vi "IV(H)_2devices_DC_temperature sweep_BF_LD-400_K6221_K2182A_PK.vi"() -> ()   [LabVIEW 2016]
uses:
  <vilib>/Math Plots/2D Math Plots/2D Compass/2D Compass XCtrl/2D Compass.xctl
  <vilib>/Math Plots/2D Math Plots/2D Compass/2D Compass Datatype/2D Compass Datatype.lvclass
  <vilib>/Math Plots/2D Math Plots/2D Compass/2D Compass Datatype/Public/Plot Helper (Vector).vi
  Labview Drivers/Keithley 622x LV 2009/Keithley 622x.lvlib
panel:
  out "data 2":dbl[](array[numeric])=[0.5999981386233562, 330.0003030452058, -2e-06, -1.74783916e-05, 8.739195800000001, 14115.23]
  out "File path 2":path=path "D:/Pranava/Data/PtTe2/29-10-2022/002/025_29-10-2022_002_DevD2_I_39-36_V_42-41_DC_IV(H)_baseT_[450mT_to_-650mT]_IP_[150deg]_10mT_steps.dat"
  in  "Measure two devices?":bool
  out "2D Compass":refnum<class "2D Plot Datatype.lvclass">[](xcontrol)
  in  "Number Averaging":i32=1
  in  "Tab Control":enum32{"Device 1", "Device 2"}(tab)=enum."Device 2"
  out "V vs I":cluster{dbl, "Field Reading":dbl}[](graph)=[{0.0, "Field Reading"=4.40241798e-08}, {2e-08, "Field Reading"=1.23783257e-07}, {4e-08, "Field Reading"=3.02986118e-07}, {6e-08, "Field Reading"=5.49519534e-07}, {8e-08, "Field Reading"=7.0386157e-07}, {1e-07, "Field Reading"=8.50435e-07}, {1.2e-07, "Field Reading"=1.09593255e-06}, {1.4e-07, "Field Reading"=1.21350074e-06}, {1.6e-07, "Field Reading"=1.39529319e-06}, {1.8e-07, "Field Reading"=1.54134866e-06}, {2e-07, "Field Reading"=1.75991058e-06}, {2.2e-07, "Field Reading"=1.91891414e-06}, {2.4e-07, "Field Reading"=2.05875441e-06}, {2.6e-07, "Field Reading"=2.23173979e-06}, {2.8e-07, "Field Reading"=2.36018563e-06}, {3e-07, "Field Reading"=2.64452742e-06}, {3.2e-07, "Field Reading"=2.75122088e-06}, {3.4e-07, "Field Reading"=2.90763477e-06}, {3.6e-07, "Field Reading"=3.12050268e-06}, {3.8e-07, "Field Reading"=3.23392292e-06}, {4e-07, "Field Reading"=3.48200967e-06}, {4.2e-07, "Field Reading"=3.63013662e-06}, {4.4e-07, "Field Reading"=3.79483537e-06}, {4.6e-07, "Field Reading"=3.94296229e-06}, {4.8e-07, "Field Reading"=4.10869871e-06}, {5e-07, "Field Reading"=4.332443e-06}, {5.2e-07, "Field Reading"=4.44638679e-06}, {5.4e-07, "Field Reading"=4.61160528e-06}, {5.6e-07, "Field Reading"=4.8415635e-06}, {5.8e-07, "Field Reading"=4.99228004e-06}, {6e-07, "Field Reading"=5.17562593e-06}, {6.2e-07, "Field Reading"=5.33774246e-06}, {6.4e-07, "Field Reading"=5.53403662e-06}, {6.6e-07, "Field Reading"=5.65315972e-06}, {6.8e-07, "Field Reading"=5.83340484e-06}, {7e-07, "Field Reading"=6.04161144e-06}, {7.2e-07, "Field Reading"=6.14312511e-06}, {7.4e-07, "Field Reading"=6.37827086e-06}, {7.6e-07, "Field Reading"=6.53727451e-06}, {7.8e-07, "Field Reading"=6.69938572e-06}, {8e-07, "Field Reading"=6.88635475e-06}, {8.2e-07, "Field Reading"=7.02101579e-06}, {8.4e-07, "Field Reading"=7.23699138e-06}, {8.6e-07, "Field Reading"=7.41308471e-06}, {8.8e-07, "Field Reading"=7.58244684e-06}, {9e-07, "Field Reading"=7.74041457e-06}, {9.2e-07, "Field Reading"=7.90562381e-06}, {9.4e-07, "Field Reading"=8.06618106e-06}, {9.6e-07, "Field Reading"=8.2422761e-06}, {9.8e-07, "Field Reading"=8.41162272e-06}, {1e-06, "Field Reading"=8.59082511e-06}, {1.02e-06, "Field Reading"=8.73842623e-06}, {1.04e-06, "Field Reading"=8.94248895e-06}, {1.06e-06, "Field Reading"=9.14240827e-06}, {1.08e-06, "Field Reading"=9.27862314e-06}, {1.1e-06, "Field Reading"=9.47388113e-06}, {1.12e-06, "Field Reading"=9.62770506e-06}, {1.14e-06, "Field Reading"=9.81261485e-06}, {1.16e-06, "Field Reading"=9.94365015e-06}, {1.18e-06, "Field Reading"=1.0168948e-05}, {1.2e-06, "Field Reading"=1.03238199e-05}, {1.22e-06, "Field Reading"=1.05263292e-05}, {1.24e-06, "Field Reading"=1.0654257e-05}, {1.26e-06, "Field Reading"=1.08365675e-05}, {1.28e-06, "Field Reading"=1.09608698e-05}, {1.3e-06, "Field Reading"=1.11291959e-05}, {1.32e-06, "Field Reading"=1.13104759e-05}, {1.34e-06, "Field Reading"=1.14658539e-05}, {1.36e-06, "Field Reading"=1.17056539e-05}, {1.38e-06, "Field Reading"=1.1880715e-05}, {1.4e-06, "Field Reading"=1.20252166e-05}, {1.42e-06, "Field Reading"=1.22121882e-05}, {1.44e-06, "Field Reading"=1.23541037e-05}, {1.46e-06, "Field Reading"=1.2493426e-05}, {1.48e-06, "Field Reading"=1.27368517e-05}, {1.5e-06, "Field Reading"=1.28668613e-05}, {1.52e-06, "Field Reading"=1.3010845e-05}, {1.54e-06, "Field Reading"=1.31729562e-05}, {1.56e-06, "Field Reading"=1.34153398e-05}, {1.58e-06, "Field Reading"=1.3541714e-05}, {1.6e-06, "Field Reading"=1.36877694e-05}, {1.62e-06, "Field Reading"=1.38659327e-05}, {1.64e-06, "Field Reading"=1.40705138e-05}, {1.66e-06, "Field Reading"=1.42554137e-05}, {1.68e-06, "Field Reading"=1.43978348e-05}, {1.7e-06, "Field Reading"=1.45537307e-05}, {1.72e-06, "Field Reading"=1.4763491e-05}, {1.74e-06, "Field Reading"=1.49478731e-05}, {1.76e-06, "Field Reading"=1.50571556e-05}, {1.78e-06, "Field Reading"=1.5244645e-05}, {1.8e-06, "Field Reading"=1.54171202e-05}, {1.82e-06, "Field Reading"=1.55590321e-05}, {1.84e-06, "Field Reading"=1.57708642e-05}, {1.86e-06, "Field Reading"=1.59593796e-05}, {1.88e-06, "Field Reading"=1.60826461e-05}, {1.9e-06, "Field Reading"=1.62836016e-05}, {1.92e-06, "Field Reading"=1.64534904e-05}, {1.94e-06, "Field Reading"=1.65871155e-05}, {1.96e-06, "Field Reading"=1.68072344e-05}, {1.98e-06, "Field Reading"=1.69807332e-05}, {2e-06, "Field Reading"=1.71039997e-05}, {2.02e-06, "Field Reading"=1.73298157e-05}, {2.04e-06, "Field Reading"=1.75338777e-05}, {2.06e-06, "Field Reading"=1.76706104e-05}, {2.08e-06, "Field Reading"=1.78063071e-05}, {2.1e-06, "Field Reading"=1.79881126e-05}, {2.12e-06, "Field Reading"=1.81730125e-05}, {2.14e-06, "Field Reading"=1.83542869e-05}, {2.16e-06, "Field Reading"=1.84765118e-05}, {2.18e-06, "Field Reading"=1.86950769e-05}, {2.2e-06, "Field Reading"=1.88804946e-05}, {2.22e-06, "Field Reading"=1.90384784e-05}, {2.24e-06, "Field Reading"=1.91767649e-05}, {2.26e-06, "Field Reading"=1.93580394e-05}, {2.28e-06, "Field Reading"=1.95553725e-05}, {2.3e-06, "Field Reading"=1.97330215e-05}, {2.32e-06, "Field Reading"=1.98827024e-05}, {2.34e-06, "Field Reading"=2.00670785e-05}, {2.36e-06, "Field Reading"=2.02561219e-05}, {2.38e-06, "Field Reading"=2.04550059e-05}, {2.4e-06, "Field Reading"=2.05839566e-05}, {2.42e-06, "Field Reading"=2.07004901e-05}, {2.44e-06, "Field Reading"=2.08941947e-05}, {2.46e-06, "Field Reading"=2.10935914e-05}, {2.48e-06, "Field Reading"=2.12541486e-05}, {2.5e-06, "Field Reading"=2.14209052e-05}, {2.52e-06, "Field Reading"=2.16146097e-05}, {2.54e-06, "Field Reading"=2.18026169e-05}, {2.56e-06, "Field Reading"=2.19916641e-05}, {2.58e-06, "Field Reading"=2.21568827e-05}, {2.6e-06, "Field Reading"=2.23319418e-05}, {2.62e-06, "Field Reading"=2.2459882e-05}, {2.64e-06, "Field Reading"=2.26406384e-05}, {2.66e-06, "Field Reading"=2.28395223e-05}, {2.68e-06, "Field Reading"=2.2994903e-05}, {2.7e-06, "Field Reading"=2.31471734e-05}, {2.72e-06, "Field Reading"=2.32978901e-05}, {2.74e-06, "Field Reading"=2.34921259e-05}, {2.76e-06, "Field Reading"=2.36547549e-05}, {2.78e-06, "Field Reading"=2.38215274e-05}, {2.8e-06, "Field Reading"=2.40152458e-05}, {2.82e-06, "Field Reading"=2.41934127e-05}, {2.84e-06, "Field Reading"=2.43938505e-05}, {2.86e-06, "Field Reading"=2.4514533e-05}, {2.88e-06, "Field Reading"=2.47548513e-05}, {2.9e-06, "Field Reading"=2.48532575e-05}, {2.92e-06, "Field Reading"=2.50619679e-05}, {2.94e-06, "Field Reading"=2.51930034e-05}, {2.96e-06, "Field Reading"=2.5380493e-05}, {2.98e-06, "Field Reading"=2.55322419e-05}, {3e-06, "Field Reading"=2.57492533e-05}, {3e-06, "Field Reading"=2.57720421e-05}, {2e-06, "Field Reading"=1.71412944e-05}, {1e-06, "Field Reading"=8.50279535e-06}, {0.0, "Field Reading"=-1.17576765e-07}, {-2e-08, "Field Reading"=-2.68811351e-07}, {-4e-08, "Field Reading"=-4.69766897e-07}, {-6e-08, "Field Reading"=-6.21518846e-07}, {-8e-08, "Field Reading"=-8.17295154e-07}, {-1e-07, "Field Reading"=-9.41079645e-07}, {-1.2e-07, "Field Reading"=-1.18502315e-06}, {-1.4e-07, "Field Reading"=-1.34454459e-06}, {-1.6e-07, "Field Reading"=-1.46573945e-06}, {-1.8e-07, "Field Reading"=-1.69051911e-06}, {-2e-07, "Field Reading"=-1.82621594e-06}, {-2.2e-07, "Field Reading"=-2.0126696e-06}, {-2.4e-07, "Field Reading"=-2.21776914e-06}, {-2.6e-07, "Field Reading"=-2.35450179e-06}, {-2.8e-07, "Field Reading"=-2.58601504e-06}, {-3e-07, "Field Reading"=-2.69322674e-06}, {-3.2e-07, "Field Reading"=-2.83721031e-06}, {-3.4e-07, "Field Reading"=-3.08995843e-06}, {-3.6e-07, "Field Reading"=-3.19457944e-06}, {-3.8e-07, "Field Reading"=-3.37844337e-06}, {-4e-07, "Field Reading"=-3.57266625e-06}, {-4.2e-07, "Field Reading"=-3.76792448e-06}, {-4.4e-07, "Field Reading"=-3.93469675e-06}, {-4.6e-07, "Field Reading"=-4.04864062e-06}, {-4.8e-07, "Field Reading"=-4.20505435e-06}, {-5e-07, "Field Reading"=-4.46867881e-06}, {-5.2e-07, "Field Reading"=-4.63596869e-06}, {-5.4e-07, "Field Reading"=-4.79238132e-06}, {-5.6e-07, "Field Reading"=-4.99799659e-06}, {-5.8e-07, "Field Reading"=-5.13783554e-06}, {-6e-07, "Field Reading"=-5.31133956e-06}, {-6.2e-07, "Field Reading"=-5.45014278e-06}, {-6.4e-07, "Field Reading"=-5.69460221e-06}, {-6.6e-07, "Field Reading"=-5.77436228e-06}, {-6.8e-07, "Field Reading"=-5.97428035e-06}, {-7e-07, "Field Reading"=-6.12913905e-06}, {-7.2e-07, "Field Reading"=-6.38136727e-06}, {-7.4e-07, "Field Reading"=-6.52534971e-06}, {-7.6e-07, "Field Reading"=-6.63359599e-06}, {-7.8e-07, "Field Reading"=-6.85112346e-06}, {-8e-07, "Field Reading"=-7.07020515e-06}, {-8.2e-07, "Field Reading"=-7.20641881e-06}, {-8.4e-07, "Field Reading"=-7.40167564e-06}, {-8.6e-07, "Field Reading"=-7.54669386e-06}, {-8.8e-07, "Field Reading"=-7.71035741e-06}, {-9e-07, "Field Reading"=-7.89525579e-06}, {-9.2e-07, "Field Reading"=-8.04286623e-06}, {-9.4e-07, "Field Reading"=-8.20031482e-06}, {-9.6e-07, "Field Reading"=-8.37226526e-06}, {-9.8e-07, "Field Reading"=-8.56441587e-06}, {-1e-06, "Field Reading"=-8.75760121e-06}, {-1.02e-06, "Field Reading"=-8.97305724e-06}, {-1.04e-06, "Field Reading"=-9.09994792e-06}, {-1.06e-06, "Field Reading"=-9.267755e-06}, {-1.08e-06, "Field Reading"=-9.48372893e-06}, {-1.1e-06, "Field Reading"=-9.64739249e-06}, {-1.12e-06, "Field Reading"=-9.79396472e-06}, {-1.14e-06, "Field Reading"=-9.97938118e-06}, {-1.16e-06, "Field Reading"=-1.00990192e-05}, {-1.18e-06, "Field Reading"=-1.03647137e-05}, {-1.2e-06, "Field Reading"=-1.04952302e-05}, {-1.22e-06, "Field Reading"=-1.06247112e-05}, {-1.24e-06, "Field Reading"=-1.08479359e-05}, {-1.26e-06, "Field Reading"=-1.10452646e-05}, {-1.28e-06, "Field Reading"=-1.11291712e-05}, {-1.3e-06, "Field Reading"=-1.13979733e-05}, {-1.32e-06, "Field Reading"=-1.15290079e-05}, {-1.34e-06, "Field Reading"=-1.17107996e-05}, {-1.36e-06, "Field Reading"=-1.18584077e-05}, {-1.38e-06, "Field Reading"=-1.2031394e-05}, {-1.4e-06, "Field Reading"=-1.22214705e-05}, {-1.42e-06, "Field Reading"=-1.23742578e-05}, {-1.44e-06, "Field Reading"=-1.25384394e-05}, {-1.46e-06, "Field Reading"=-1.27621798e-05}, {-1.48e-06, "Field Reading"=-1.28792304e-05}, {-1.5e-06, "Field Reading"=-1.30289101e-05}, {-1.52e-06, "Field Reading"=-1.32428105e-05}, {-1.54e-06, "Field Reading"=-1.34660352e-05}, {-1.56e-06, "Field Reading"=-1.35644406e-05}, {-1.58e-06, "Field Reading"=-1.37255157e-05}, {-1.6e-06, "Field Reading"=-1.39409717e-05}, {-1.62e-06, "Field Reading"=-1.41439974e-05}, {-1.64e-06, "Field Reading"=-1.42952297e-05}, {-1.66e-06, "Field Reading"=-1.44941121e-05}, {-1.68e-06, "Field Reading"=-1.45919995e-05}, {-1.7e-06, "Field Reading"=-1.47965808e-05}, {-1.72e-06, "Field Reading"=-1.50275744e-05}, {-1.74e-06, "Field Reading"=-1.51088883e-05}, {-1.76e-06, "Field Reading"=-1.5286534e-05}, {-1.78e-06, "Field Reading"=-1.55475671e-05}, {-1.8e-06, "Field Reading"=-1.56418291e-05}, {-1.82e-06, "Field Reading"=-1.58401957e-05}, {-1.84e-06, "Field Reading"=-1.60354527e-05}, {-1.86e-06, "Field Reading"=-1.61778815e-05}, {-1.88e-06, "Field Reading"=-1.64109433e-05}, {-1.9e-06, "Field Reading"=-1.65114203e-05}, {-1.92e-06, "Field Reading"=-1.67460393e-05}, {-1.94e-06, "Field Reading"=-1.69164354e-05}, {-1.96e-06, "Field Reading"=-1.7107031e-05}, {-1.98e-06, "Field Reading"=-1.72157948e-05}, {-2e-06, "Field Reading"=-1.73789424e-05}, {-2.02e-06, "Field Reading"=-1.7616151e-05}, {-2.04e-06, "Field Reading"=-1.77135205e-05}, {-2.06e-06, "Field Reading"=-1.788599e-05}, {-2.08e-06, "Field Reading"=-1.80781394e-05}, {-2.1e-06, "Field Reading"=-1.82045126e-05}, {-2.12e-06, "Field Reading"=-1.84603712e-05}, {-2.14e-06, "Field Reading"=-1.8589852e-05}, {-2.16e-06, "Field Reading"=-1.87690534e-05}, {-2.18e-06, "Field Reading"=-1.89917572e-05}, {-2.2e-06, "Field Reading"=-1.91388473e-05}, {-2.22e-06, "Field Reading"=-1.93584466e-05}, {-2.24e-06, "Field Reading"=-1.95366097e-05}, {-2.26e-06, "Field Reading"=-1.96655725e-05}, {-2.28e-06, "Field Reading"=-1.98468455e-05}, {-2.3e-06, "Field Reading"=-2.00260392e-05}, {-2.32e-06, "Field Reading"=-2.02104196e-05}, {-2.34e-06, "Field Reading"=-2.03642427e-05}, {-2.36e-06, "Field Reading"=-2.05486354e-05}, {-2.38e-06, "Field Reading"=-2.07009048e-05}, {-2.4e-06, "Field Reading"=-2.08485128e-05}, {-2.42e-06, "Field Reading"=-2.10551707e-05}, {-2.44e-06, "Field Reading"=-2.12468023e-05}, {-2.46e-06, "Field Reading"=-2.14161632e-05}, {-2.48e-06, "Field Reading"=-2.1574128e-05}, {-2.5e-06, "Field Reading"=-2.17181107e-05}, {-2.52e-06, "Field Reading"=-2.18755593e-05}, {-2.54e-06, "Field Reading"=-2.21179489e-05}, {-2.56e-06, "Field Reading"=-2.22878278e-05}, {-2.58e-06, "Field Reading"=-2.246185e-05}, {-2.6e-06, "Field Reading"=-2.26146323e-05}, {-2.62e-06, "Field Reading"=-2.28161044e-05}, {-2.64e-06, "Field Reading"=-2.29424776e-05}, {-2.66e-06, "Field Reading"=-2.30880191e-05}, {-2.68e-06, "Field Reading"=-2.32863837e-05}, {-2.7e-06, "Field Reading"=-2.34681748e-05}, {-2.72e-06, "Field Reading"=-2.36484132e-05}, {-2.74e-06, "Field Reading"=-2.38566183e-05}, {-2.76e-06, "Field Reading"=-2.39985293e-05}, {-2.78e-06, "Field Reading"=-2.41513117e-05}, {-2.8e-06, "Field Reading"=-2.43227442e-05}, {-2.82e-06, "Field Reading"=-2.44646552e-05}, {-2.84e-06, "Field Reading"=-2.46112313e-05}, {-2.86e-06, "Field Reading"=-2.47919865e-05}, {-2.88e-06, "Field Reading"=-2.50271236e-05}, {-2.9e-06, "Field Reading"=-2.51327718e-05}, {-2.92e-06, "Field Reading"=-2.53295825e-05}, {-2.94e-06, "Field Reading"=-2.55269109e-05}, {-2.96e-06, "Field Reading"=-2.57024868e-05}, {-2.98e-06, "Field Reading"=-2.5883242e-05}, {-3e-06, "Field Reading"=-2.59930485e-05}, {-3e-06, "Field Reading"=-2.60981869e-05}, {-2e-06, "Field Reading"=-1.74783916e-05}]
  in  "File name 1":string="027_29-10-2022_002_DevH3_I_46-48_V_45-43_DC_IV(H)_baseT_[-600mT_to_600mT]_IP_[146deg]_5mT_steps"
  in  "From 3":dbl[](array[numeric])=[0.0, 0.00032, 0.0, -0.00032] min=-3000.0 max=3000.0 format="%.1e"
  in  "To 3":dbl[](array[numeric])=[0.00032, 1e-06, -0.00032, -1e-06] min=-3000.0 max=3000.0 format="%.1e"
  in  "Step 3":dbl[](array[numeric])=[2e-06, 0.0001, 2e-06, 1e-06] min=-3000.0 max=3000.0 format="%.1e"
  in  "Current source K6221 VISA Device 1":refnum<visa-resource-name>="GPIB0::13::INSTR"
  in  "Nanovoltmeter 2182a VISA Device1":refnum<visa-resource-name>="GPIB0::7::INSTR"
  in  "wait (ms)":u32=50
  in  "Set Compliance voltage (V)":dbl=5.0 min=0.0 step=0.1 format="%_3f"
  out "Resistance (ohm)":dbl=8.739195800000001 format="%#_13g"
  out "Time (s)":dbl=14115.488 format="%#_13g"
  out "Iset (A)":dbl=-2e-06
  out "Vmeas (V)":dbl=-1.74783916e-05
  in  "File name 2":string="027_29-10-2022_002_DevH3_I_46-48_V_45-43_DC_IV(H)_baseT_[-600mT_to_600mT]_IP_[146deg]_5mT_steps"
  in  "Current source K6221 VISA Device 2":refnum<visa-resource-name>="GPIB0::13::INSTR"
  in  "Nanovoltmeter 2182a VISA Device 2":refnum<visa-resource-name>="GPIB0::7::INSTR"
  in  "Set Compliance voltage (V) 2":dbl=5.0 min=0.0 step=0.1 format="%_3f"
  in  "wait (ms) 2":u32=50
  in  "To 4":dbl[](array[numeric])=[0.00032, 1e-06, -0.00032, -1e-06] min=-3000.0 max=3000.0 format="%.1e"
  in  "From 4":dbl[](array[numeric])=[0.0, 0.00032, 0.0, -0.00032] min=-3000.0 max=3000.0 format="%.1e"
  in  "Step 4":dbl[](array[numeric])=[2e-06, 0.0001, 2e-06, 1e-06] min=-3000.0 max=3000.0 format="%.1e"
  out "V vs I 2":cluster{dbl, "Field Reading":dbl}[](graph)=[{0.0, "Field Reading"=4.40241798e-08}, {2e-08, "Field Reading"=1.23783257e-07}, {4e-08, "Field Reading"=3.02986118e-07}, {6e-08, "Field Reading"=5.49519534e-07}, {8e-08, "Field Reading"=7.0386157e-07}, {1e-07, "Field Reading"=8.50435e-07}, {1.2e-07, "Field Reading"=1.09593255e-06}, {1.4e-07, "Field Reading"=1.21350074e-06}, {1.6e-07, "Field Reading"=1.39529319e-06}, {1.8e-07, "Field Reading"=1.54134866e-06}, {2e-07, "Field Reading"=1.75991058e-06}, {2.2e-07, "Field Reading"=1.91891414e-06}, {2.4e-07, "Field Reading"=2.05875441e-06}, {2.6e-07, "Field Reading"=2.23173979e-06}, {2.8e-07, "Field Reading"=2.36018563e-06}, {3e-07, "Field Reading"=2.64452742e-06}, {3.2e-07, "Field Reading"=2.75122088e-06}, {3.4e-07, "Field Reading"=2.90763477e-06}, {3.6e-07, "Field Reading"=3.12050268e-06}, {3.8e-07, "Field Reading"=3.23392292e-06}, {4e-07, "Field Reading"=3.48200967e-06}, {4.2e-07, "Field Reading"=3.63013662e-06}, {4.4e-07, "Field Reading"=3.79483537e-06}, {4.6e-07, "Field Reading"=3.94296229e-06}, {4.8e-07, "Field Reading"=4.10869871e-06}, {5e-07, "Field Reading"=4.332443e-06}, {5.2e-07, "Field Reading"=4.44638679e-06}, {5.4e-07, "Field Reading"=4.61160528e-06}, {5.6e-07, "Field Reading"=4.8415635e-06}, {5.8e-07, "Field Reading"=4.99228004e-06}, {6e-07, "Field Reading"=5.17562593e-06}, {6.2e-07, "Field Reading"=5.33774246e-06}, {6.4e-07, "Field Reading"=5.53403662e-06}, {6.6e-07, "Field Reading"=5.65315972e-06}, {6.8e-07, "Field Reading"=5.83340484e-06}, {7e-07, "Field Reading"=6.04161144e-06}, {7.2e-07, "Field Reading"=6.14312511e-06}, {7.4e-07, "Field Reading"=6.37827086e-06}, {7.6e-07, "Field Reading"=6.53727451e-06}, {7.8e-07, "Field Reading"=6.69938572e-06}, {8e-07, "Field Reading"=6.88635475e-06}, {8.2e-07, "Field Reading"=7.02101579e-06}, {8.4e-07, "Field Reading"=7.23699138e-06}, {8.6e-07, "Field Reading"=7.41308471e-06}, {8.8e-07, "Field Reading"=7.58244684e-06}, {9e-07, "Field Reading"=7.74041457e-06}, {9.2e-07, "Field Reading"=7.90562381e-06}, {9.4e-07, "Field Reading"=8.06618106e-06}, {9.6e-07, "Field Reading"=8.2422761e-06}, {9.8e-07, "Field Reading"=8.41162272e-06}, {1e-06, "Field Reading"=8.59082511e-06}, {1.02e-06, "Field Reading"=8.73842623e-06}, {1.04e-06, "Field Reading"=8.94248895e-06}, {1.06e-06, "Field Reading"=9.14240827e-06}, {1.08e-06, "Field Reading"=9.27862314e-06}, {1.1e-06, "Field Reading"=9.47388113e-06}, {1.12e-06, "Field Reading"=9.62770506e-06}, {1.14e-06, "Field Reading"=9.81261485e-06}, {1.16e-06, "Field Reading"=9.94365015e-06}, {1.18e-06, "Field Reading"=1.0168948e-05}, {1.2e-06, "Field Reading"=1.03238199e-05}, {1.22e-06, "Field Reading"=1.05263292e-05}, {1.24e-06, "Field Reading"=1.0654257e-05}, {1.26e-06, "Field Reading"=1.08365675e-05}, {1.28e-06, "Field Reading"=1.09608698e-05}, {1.3e-06, "Field Reading"=1.11291959e-05}, {1.32e-06, "Field Reading"=1.13104759e-05}, {1.34e-06, "Field Reading"=1.14658539e-05}, {1.36e-06, "Field Reading"=1.17056539e-05}, {1.38e-06, "Field Reading"=1.1880715e-05}, {1.4e-06, "Field Reading"=1.20252166e-05}, {1.42e-06, "Field Reading"=1.22121882e-05}, {1.44e-06, "Field Reading"=1.23541037e-05}, {1.46e-06, "Field Reading"=1.2493426e-05}, {1.48e-06, "Field Reading"=1.27368517e-05}, {1.5e-06, "Field Reading"=1.28668613e-05}, {1.52e-06, "Field Reading"=1.3010845e-05}, {1.54e-06, "Field Reading"=1.31729562e-05}, {1.56e-06, "Field Reading"=1.34153398e-05}, {1.58e-06, "Field Reading"=1.3541714e-05}, {1.6e-06, "Field Reading"=1.36877694e-05}, {1.62e-06, "Field Reading"=1.38659327e-05}, {1.64e-06, "Field Reading"=1.40705138e-05}, {1.66e-06, "Field Reading"=1.42554137e-05}, {1.68e-06, "Field Reading"=1.43978348e-05}, {1.7e-06, "Field Reading"=1.45537307e-05}, {1.72e-06, "Field Reading"=1.4763491e-05}, {1.74e-06, "Field Reading"=1.49478731e-05}, {1.76e-06, "Field Reading"=1.50571556e-05}, {1.78e-06, "Field Reading"=1.5244645e-05}, {1.8e-06, "Field Reading"=1.54171202e-05}, {1.82e-06, "Field Reading"=1.55590321e-05}, {1.84e-06, "Field Reading"=1.57708642e-05}, {1.86e-06, "Field Reading"=1.59593796e-05}, {1.88e-06, "Field Reading"=1.60826461e-05}, {1.9e-06, "Field Reading"=1.62836016e-05}, {1.92e-06, "Field Reading"=1.64534904e-05}, {1.94e-06, "Field Reading"=1.65871155e-05}, {1.96e-06, "Field Reading"=1.68072344e-05}, {1.98e-06, "Field Reading"=1.69807332e-05}, {2e-06, "Field Reading"=1.71039997e-05}, {2.02e-06, "Field Reading"=1.73298157e-05}, {2.04e-06, "Field Reading"=1.75338777e-05}, {2.06e-06, "Field Reading"=1.76706104e-05}, {2.08e-06, "Field Reading"=1.78063071e-05}, {2.1e-06, "Field Reading"=1.79881126e-05}, {2.12e-06, "Field Reading"=1.81730125e-05}, {2.14e-06, "Field Reading"=1.83542869e-05}, {2.16e-06, "Field Reading"=1.84765118e-05}, {2.18e-06, "Field Reading"=1.86950769e-05}, {2.2e-06, "Field Reading"=1.88804946e-05}, {2.22e-06, "Field Reading"=1.90384784e-05}, {2.24e-06, "Field Reading"=1.91767649e-05}, {2.26e-06, "Field Reading"=1.93580394e-05}, {2.28e-06, "Field Reading"=1.95553725e-05}, {2.3e-06, "Field Reading"=1.97330215e-05}, {2.32e-06, "Field Reading"=1.98827024e-05}, {2.34e-06, "Field Reading"=2.00670785e-05}, {2.36e-06, "Field Reading"=2.02561219e-05}, {2.38e-06, "Field Reading"=2.04550059e-05}, {2.4e-06, "Field Reading"=2.05839566e-05}, {2.42e-06, "Field Reading"=2.07004901e-05}, {2.44e-06, "Field Reading"=2.08941947e-05}, {2.46e-06, "Field Reading"=2.10935914e-05}, {2.48e-06, "Field Reading"=2.12541486e-05}, {2.5e-06, "Field Reading"=2.14209052e-05}, {2.52e-06, "Field Reading"=2.16146097e-05}, {2.54e-06, "Field Reading"=2.18026169e-05}, {2.56e-06, "Field Reading"=2.19916641e-05}, {2.58e-06, "Field Reading"=2.21568827e-05}, {2.6e-06, "Field Reading"=2.23319418e-05}, {2.62e-06, "Field Reading"=2.2459882e-05}, {2.64e-06, "Field Reading"=2.26406384e-05}, {2.66e-06, "Field Reading"=2.28395223e-05}, {2.68e-06, "Field Reading"=2.2994903e-05}, {2.7e-06, "Field Reading"=2.31471734e-05}, {2.72e-06, "Field Reading"=2.32978901e-05}, {2.74e-06, "Field Reading"=2.34921259e-05}, {2.76e-06, "Field Reading"=2.36547549e-05}, {2.78e-06, "Field Reading"=2.38215274e-05}, {2.8e-06, "Field Reading"=2.40152458e-05}, {2.82e-06, "Field Reading"=2.41934127e-05}, {2.84e-06, "Field Reading"=2.43938505e-05}, {2.86e-06, "Field Reading"=2.4514533e-05}, {2.88e-06, "Field Reading"=2.47548513e-05}, {2.9e-06, "Field Reading"=2.48532575e-05}, {2.92e-06, "Field Reading"=2.50619679e-05}, {2.94e-06, "Field Reading"=2.51930034e-05}, {2.96e-06, "Field Reading"=2.5380493e-05}, {2.98e-06, "Field Reading"=2.55322419e-05}, {3e-06, "Field Reading"=2.57492533e-05}, {3e-06, "Field Reading"=2.57720421e-05}, {2e-06, "Field Reading"=1.71412944e-05}, {1e-06, "Field Reading"=8.50279535e-06}, {0.0, "Field Reading"=-1.17576765e-07}, {-2e-08, "Field Reading"=-2.68811351e-07}, {-4e-08, "Field Reading"=-4.69766897e-07}, {-6e-08, "Field Reading"=-6.21518846e-07}, {-8e-08, "Field Reading"=-8.17295154e-07}, {-1e-07, "Field Reading"=-9.41079645e-07}, {-1.2e-07, "Field Reading"=-1.18502315e-06}, {-1.4e-07, "Field Reading"=-1.34454459e-06}, {-1.6e-07, "Field Reading"=-1.46573945e-06}, {-1.8e-07, "Field Reading"=-1.69051911e-06}, {-2e-07, "Field Reading"=-1.82621594e-06}, {-2.2e-07, "Field Reading"=-2.0126696e-06}, {-2.4e-07, "Field Reading"=-2.21776914e-06}, {-2.6e-07, "Field Reading"=-2.35450179e-06}, {-2.8e-07, "Field Reading"=-2.58601504e-06}, {-3e-07, "Field Reading"=-2.69322674e-06}, {-3.2e-07, "Field Reading"=-2.83721031e-06}, {-3.4e-07, "Field Reading"=-3.08995843e-06}, {-3.6e-07, "Field Reading"=-3.19457944e-06}, {-3.8e-07, "Field Reading"=-3.37844337e-06}, {-4e-07, "Field Reading"=-3.57266625e-06}, {-4.2e-07, "Field Reading"=-3.76792448e-06}, {-4.4e-07, "Field Reading"=-3.93469675e-06}, {-4.6e-07, "Field Reading"=-4.04864062e-06}, {-4.8e-07, "Field Reading"=-4.20505435e-06}, {-5e-07, "Field Reading"=-4.46867881e-06}, {-5.2e-07, "Field Reading"=-4.63596869e-06}, {-5.4e-07, "Field Reading"=-4.79238132e-06}, {-5.6e-07, "Field Reading"=-4.99799659e-06}, {-5.8e-07, "Field Reading"=-5.13783554e-06}, {-6e-07, "Field Reading"=-5.31133956e-06}, {-6.2e-07, "Field Reading"=-5.45014278e-06}, {-6.4e-07, "Field Reading"=-5.69460221e-06}, {-6.6e-07, "Field Reading"=-5.77436228e-06}, {-6.8e-07, "Field Reading"=-5.97428035e-06}, {-7e-07, "Field Reading"=-6.12913905e-06}, {-7.2e-07, "Field Reading"=-6.38136727e-06}, {-7.4e-07, "Field Reading"=-6.52534971e-06}, {-7.6e-07, "Field Reading"=-6.63359599e-06}, {-7.8e-07, "Field Reading"=-6.85112346e-06}, {-8e-07, "Field Reading"=-7.07020515e-06}, {-8.2e-07, "Field Reading"=-7.20641881e-06}, {-8.4e-07, "Field Reading"=-7.40167564e-06}, {-8.6e-07, "Field Reading"=-7.54669386e-06}, {-8.8e-07, "Field Reading"=-7.71035741e-06}, {-9e-07, "Field Reading"=-7.89525579e-06}, {-9.2e-07, "Field Reading"=-8.04286623e-06}, {-9.4e-07, "Field Reading"=-8.20031482e-06}, {-9.6e-07, "Field Reading"=-8.37226526e-06}, {-9.8e-07, "Field Reading"=-8.56441587e-06}, {-1e-06, "Field Reading"=-8.75760121e-06}, {-1.02e-06, "Field Reading"=-8.97305724e-06}, {-1.04e-06, "Field Reading"=-9.09994792e-06}, {-1.06e-06, "Field Reading"=-9.267755e-06}, {-1.08e-06, "Field Reading"=-9.48372893e-06}, {-1.1e-06, "Field Reading"=-9.64739249e-06}, {-1.12e-06, "Field Reading"=-9.79396472e-06}, {-1.14e-06, "Field Reading"=-9.97938118e-06}, {-1.16e-06, "Field Reading"=-1.00990192e-05}, {-1.18e-06, "Field Reading"=-1.03647137e-05}, {-1.2e-06, "Field Reading"=-1.04952302e-05}, {-1.22e-06, "Field Reading"=-1.06247112e-05}, {-1.24e-06, "Field Reading"=-1.08479359e-05}, {-1.26e-06, "Field Reading"=-1.10452646e-05}, {-1.28e-06, "Field Reading"=-1.11291712e-05}, {-1.3e-06, "Field Reading"=-1.13979733e-05}, {-1.32e-06, "Field Reading"=-1.15290079e-05}, {-1.34e-06, "Field Reading"=-1.17107996e-05}, {-1.36e-06, "Field Reading"=-1.18584077e-05}, {-1.38e-06, "Field Reading"=-1.2031394e-05}, {-1.4e-06, "Field Reading"=-1.22214705e-05}, {-1.42e-06, "Field Reading"=-1.23742578e-05}, {-1.44e-06, "Field Reading"=-1.25384394e-05}, {-1.46e-06, "Field Reading"=-1.27621798e-05}, {-1.48e-06, "Field Reading"=-1.28792304e-05}, {-1.5e-06, "Field Reading"=-1.30289101e-05}, {-1.52e-06, "Field Reading"=-1.32428105e-05}, {-1.54e-06, "Field Reading"=-1.34660352e-05}, {-1.56e-06, "Field Reading"=-1.35644406e-05}, {-1.58e-06, "Field Reading"=-1.37255157e-05}, {-1.6e-06, "Field Reading"=-1.39409717e-05}, {-1.62e-06, "Field Reading"=-1.41439974e-05}, {-1.64e-06, "Field Reading"=-1.42952297e-05}, {-1.66e-06, "Field Reading"=-1.44941121e-05}, {-1.68e-06, "Field Reading"=-1.45919995e-05}, {-1.7e-06, "Field Reading"=-1.47965808e-05}, {-1.72e-06, "Field Reading"=-1.50275744e-05}, {-1.74e-06, "Field Reading"=-1.51088883e-05}, {-1.76e-06, "Field Reading"=-1.5286534e-05}, {-1.78e-06, "Field Reading"=-1.55475671e-05}, {-1.8e-06, "Field Reading"=-1.56418291e-05}, {-1.82e-06, "Field Reading"=-1.58401957e-05}, {-1.84e-06, "Field Reading"=-1.60354527e-05}, {-1.86e-06, "Field Reading"=-1.61778815e-05}, {-1.88e-06, "Field Reading"=-1.64109433e-05}, {-1.9e-06, "Field Reading"=-1.65114203e-05}, {-1.92e-06, "Field Reading"=-1.67460393e-05}, {-1.94e-06, "Field Reading"=-1.69164354e-05}, {-1.96e-06, "Field Reading"=-1.7107031e-05}, {-1.98e-06, "Field Reading"=-1.72157948e-05}, {-2e-06, "Field Reading"=-1.73789424e-05}, {-2.02e-06, "Field Reading"=-1.7616151e-05}, {-2.04e-06, "Field Reading"=-1.77135205e-05}, {-2.06e-06, "Field Reading"=-1.788599e-05}, {-2.08e-06, "Field Reading"=-1.80781394e-05}, {-2.1e-06, "Field Reading"=-1.82045126e-05}, {-2.12e-06, "Field Reading"=-1.84603712e-05}, {-2.14e-06, "Field Reading"=-1.8589852e-05}, {-2.16e-06, "Field Reading"=-1.87690534e-05}, {-2.18e-06, "Field Reading"=-1.89917572e-05}, {-2.2e-06, "Field Reading"=-1.91388473e-05}, {-2.22e-06, "Field Reading"=-1.93584466e-05}, {-2.24e-06, "Field Reading"=-1.95366097e-05}, {-2.26e-06, "Field Reading"=-1.96655725e-05}, {-2.28e-06, "Field Reading"=-1.98468455e-05}, {-2.3e-06, "Field Reading"=-2.00260392e-05}, {-2.32e-06, "Field Reading"=-2.02104196e-05}, {-2.34e-06, "Field Reading"=-2.03642427e-05}, {-2.36e-06, "Field Reading"=-2.05486354e-05}, {-2.38e-06, "Field Reading"=-2.07009048e-05}, {-2.4e-06, "Field Reading"=-2.08485128e-05}, {-2.42e-06, "Field Reading"=-2.10551707e-05}, {-2.44e-06, "Field Reading"=-2.12468023e-05}, {-2.46e-06, "Field Reading"=-2.14161632e-05}, {-2.48e-06, "Field Reading"=-2.1574128e-05}, {-2.5e-06, "Field Reading"=-2.17181107e-05}, {-2.52e-06, "Field Reading"=-2.18755593e-05}, {-2.54e-06, "Field Reading"=-2.21179489e-05}, {-2.56e-06, "Field Reading"=-2.22878278e-05}, {-2.58e-06, "Field Reading"=-2.246185e-05}, {-2.6e-06, "Field Reading"=-2.26146323e-05}, {-2.62e-06, "Field Reading"=-2.28161044e-05}, {-2.64e-06, "Field Reading"=-2.29424776e-05}, {-2.66e-06, "Field Reading"=-2.30880191e-05}, {-2.68e-06, "Field Reading"=-2.32863837e-05}, {-2.7e-06, "Field Reading"=-2.34681748e-05}, {-2.72e-06, "Field Reading"=-2.36484132e-05}, {-2.74e-06, "Field Reading"=-2.38566183e-05}, {-2.76e-06, "Field Reading"=-2.39985293e-05}, {-2.78e-06, "Field Reading"=-2.41513117e-05}, {-2.8e-06, "Field Reading"=-2.43227442e-05}, {-2.82e-06, "Field Reading"=-2.44646552e-05}, {-2.84e-06, "Field Reading"=-2.46112313e-05}, {-2.86e-06, "Field Reading"=-2.47919865e-05}, {-2.88e-06, "Field Reading"=-2.50271236e-05}, {-2.9e-06, "Field Reading"=-2.51327718e-05}, {-2.92e-06, "Field Reading"=-2.53295825e-05}, {-2.94e-06, "Field Reading"=-2.55269109e-05}, {-2.96e-06, "Field Reading"=-2.57024868e-05}, {-2.98e-06, "Field Reading"=-2.5883242e-05}, {-3e-06, "Field Reading"=-2.59930485e-05}, {-3e-06, "Field Reading"=-2.60981869e-05}, {-2e-06, "Field Reading"=-1.74783916e-05}]
  out "Vmeas (V) 2":dbl=-1.74783916e-05
  out "Resistance (ohm) 2":dbl=8.739195800000001 format="%#_13g"
  out "Iset (A) 2":dbl=-2e-06
  out "Magnetic Field Vector Angle":dbl=330.0003030452058 format="%#_13g"
  out "Magnetic Field Vector magnitude (T)":dbl=0.5999981386233562 format="%#_13g"
  in  "From 2":dbl[](array[numeric])=[-0.6] min=-3000.0 max=3000.0 format="%#.5f"
  in  "To 2":dbl[](array[numeric])=[0.6] min=-3000.0 max=3000.0 format="%#.5g"
  in  "Step 2":dbl[](array[numeric])=[0.005] min=-3000.0 max=3000.0 format="%.5e"
  in  "Wait time after each sweep(min)":dbl=0.1 format="%#_13g"
  out "Z-axis Magnetic Field (T)":string="-0.299996321\r\n"
  in  "Y-axis Field ramp rate (T/min)":string="0.025"
  in  "Z-axis Field ramp rate (T/min)":string="0.025"
  out "Z-axis (90 deg)":dbl(slide)=-0.299996321 scale=0.0..3.0
  out "Y-Axis (0deg)":dbl(slide)=0.519615217 scale=0.0..3.0
  out "Y-axis Magnetic Field (T)":string="0.519615217\r\n"
  in  "Magnet IP Address Z-axis":string="169.254.76.2"
  in  "Magnet IP Address Y-axis":string="169.254.212.23"
  in  "Magnetic field stabilization time (s)":dbl=1.0 format="%#_13g"
  in  "Step":dbl[](array[numeric])=[1.0] min=-3000.0 max=3000.0 format="%.4g"
  in  "To":dbl[](array[numeric])=[146.37] min=-3000.0 max=3000.0 format="%.4f"
  in  "From":dbl[](array[numeric])=[146.37] min=-3000.0 max=3000.0 format="%.4f"
  in  "Folder":path=path "D:/Pranava/Data/PtTe2/29-10-2022/002"
  out "data":dbl[](array[numeric])=[0.5999981386233562, 330.0003030452058, -2e-06, -1.74783916e-05, 8.739195800000001, 14115.23]
  out "File path 1":path=path "D:/Pranava/Data/PtTe2/29-10-2022/002/025_29-10-2022_002_DevD2_I_39-36_V_42-41_DC_IV(H)_baseT_[450mT_to_-650mT]_IP_[150deg]_10mT_steps.dat"
  # "[Must be less than 0.05]"
  # "It is important that there is enough time for the magnet to cool down after each sweep (Typically 15-20 min)"
  # "Configure Field Angle (deg)"
  # "Configure Field magnitude (T)"
  # "Z-Axis: In-plane (90 deg)\nY-axis: Out-of-plane (0 deg)"
  # ".dat"
  # "Configure current sweep 1 (A)"
  # ".dat"
  # "Configure current sweep 2 (A)"
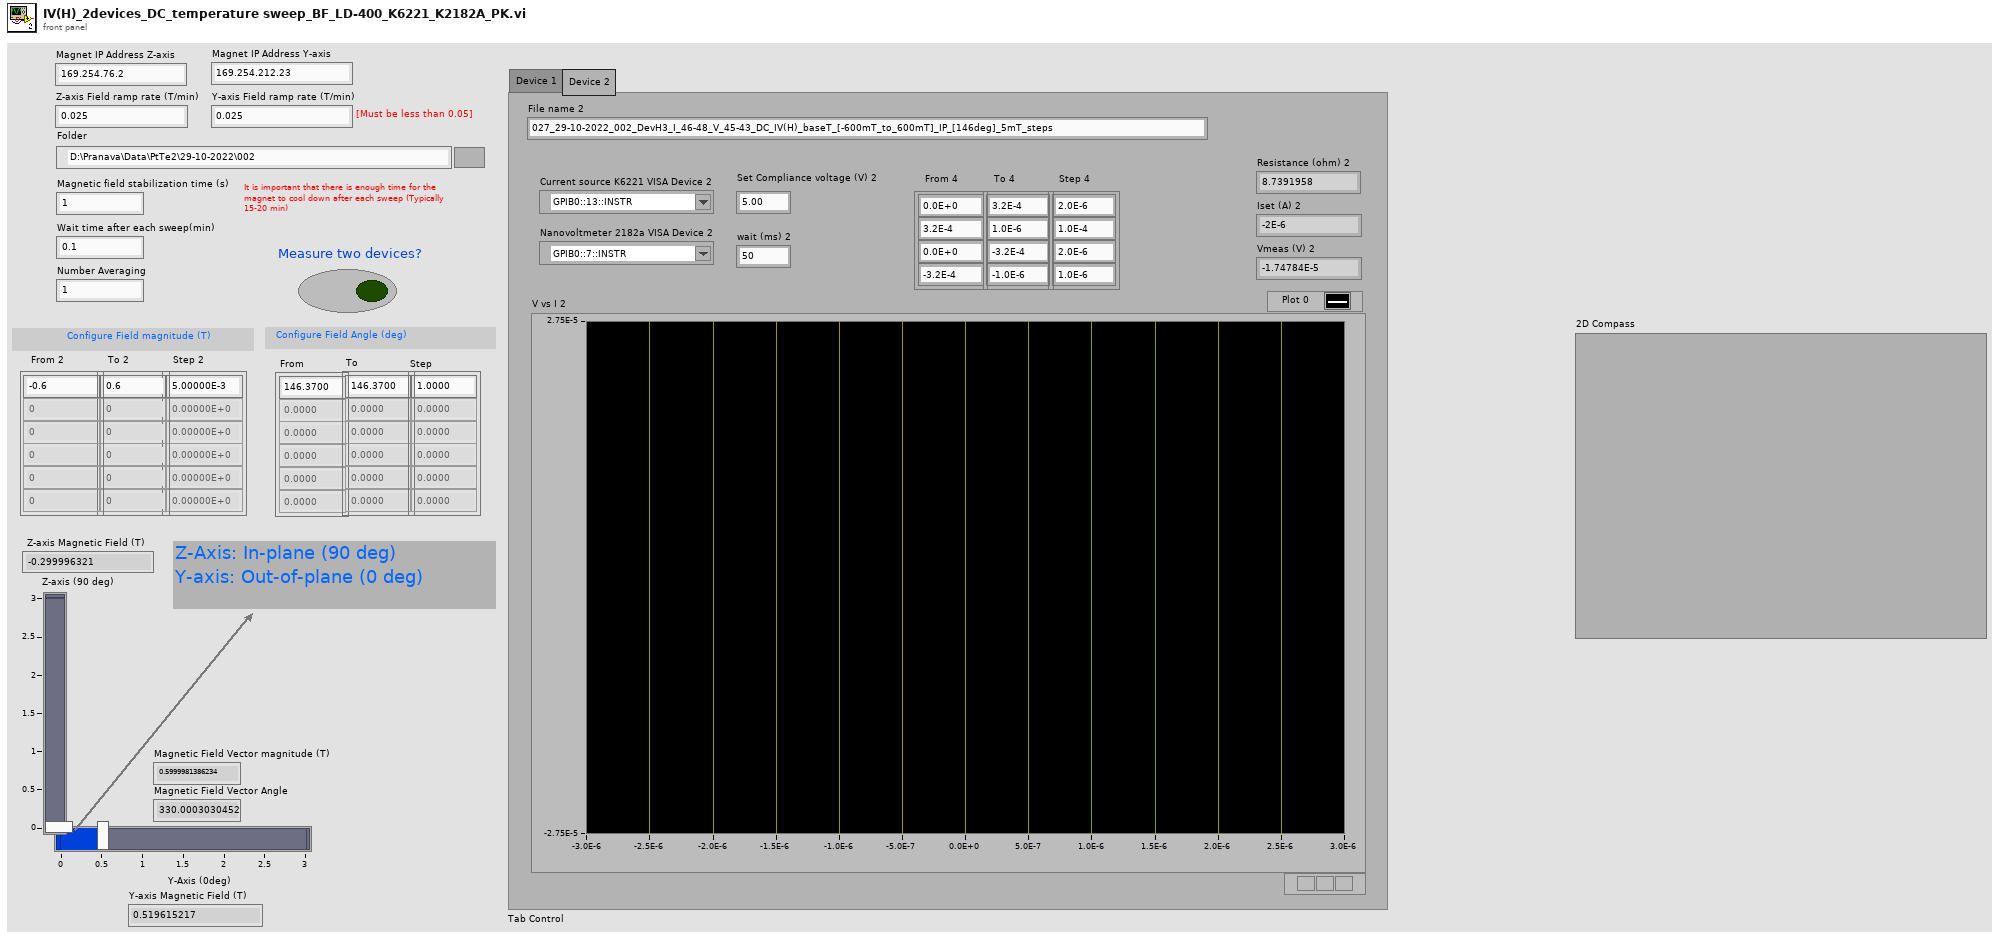
[diagram p1: front panel]
types:
  T1 = enum16{"open", "replace", "create", "open or create", "replace or create", "replace or create with confirmation"}
  T2 = typedef "Keithley 622x.lvlib/KE622x -- Current Level.ctl" = dbl
  T3 = cluster{"Average value":dbl, "Average value":dbl}
  T4 = cluster{"Average value":dbl, "Average value":dbl}[]
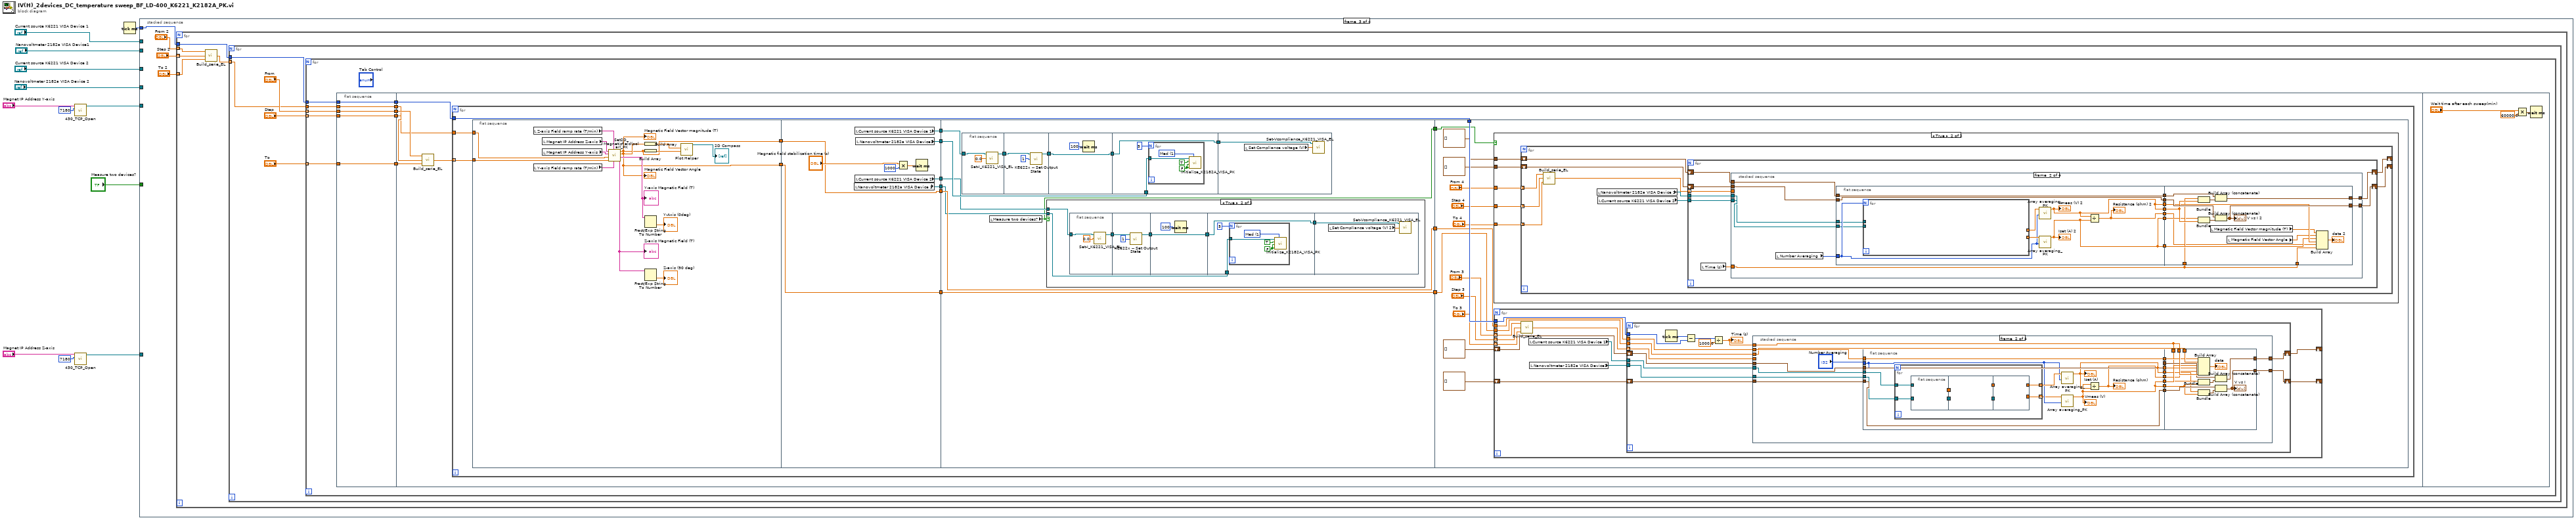
[diagram p0: block diagram]
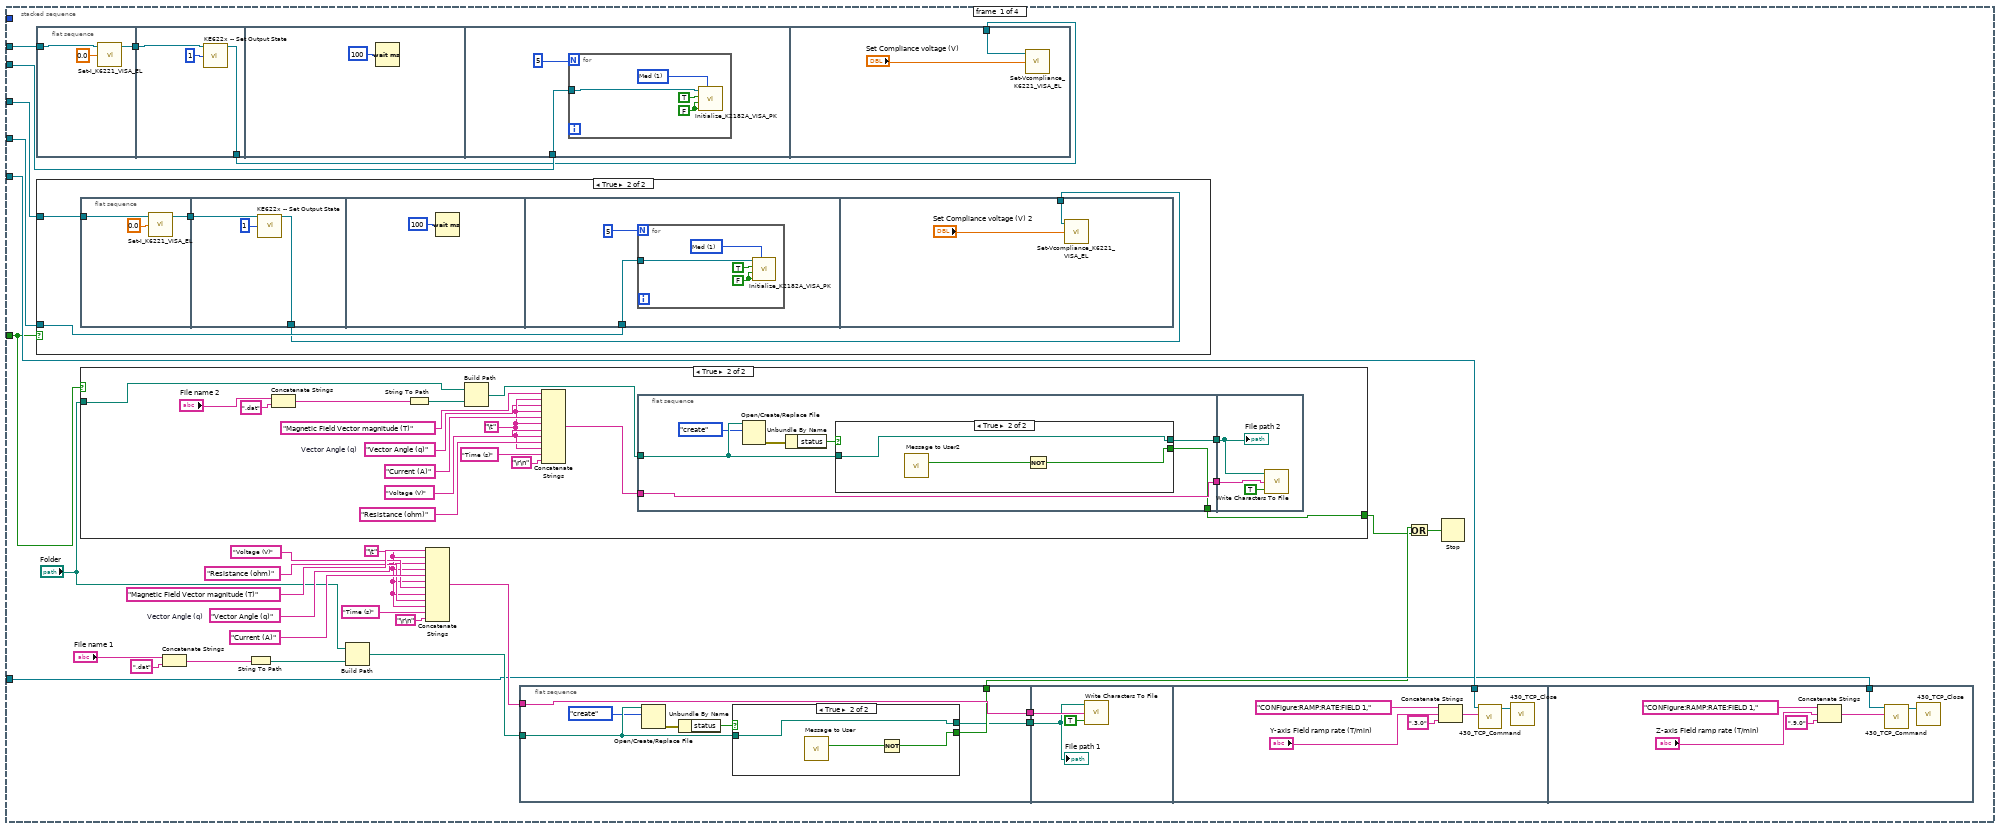
[diagram p2: hidden frame]
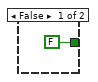
[diagram p3: hidden frame]
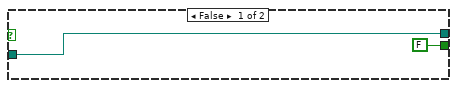
[diagram p4: hidden frame]
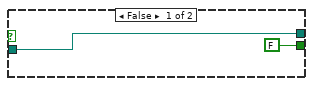
[diagram p6: hidden frame]
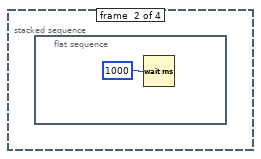
[diagram p7: hidden frame]
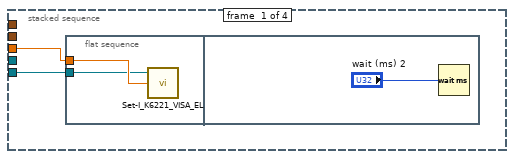
[diagram p10: hidden frame]
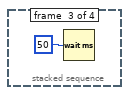
[diagram p11: hidden frame]
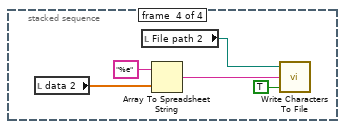
[diagram p12: hidden frame]
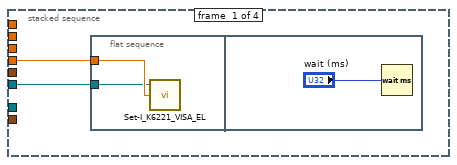
[diagram p13: hidden frame]
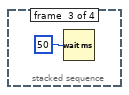
[diagram p14: hidden frame]
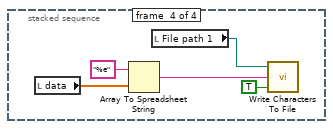
[diagram p15: hidden frame]
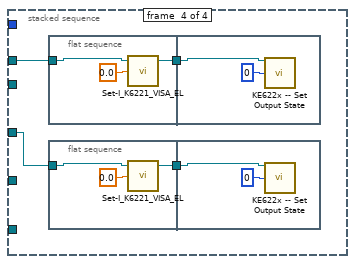
[diagram p16: hidden frame]
diagram:
  n1 = call "430_TCP_Open.vi"("IP Address"="Magnet IP Address Y-axis", "TCP Port"=7180) -> ("connection ID"=w11:refnum<k5>)  [unwired: 4 in, 2 out]
  n2 = call "430_TCP_Open.vi"("IP Address"="Magnet IP Address Z-axis", "TCP Port"=7180) -> ("connection ID"=w6:refnum<k5>)  [unwired: 4 in, 2 out]
  n3 = Tick Count (ms)() -> (millisecond timer value=w10:u32)
  n4 = stacked-sequence {
    tunnel: w11 -> [w29 _ _ _]
    tunnel: w10 -> [_ _ w141 _]
    tunnel: w6 -> [w26 _ _ _]
    tunnel: "Current source K6221 VISA Device 1" -> [w22 _ _ w473]
    tunnel: "Nanovoltmeter 2182a VISA Device1" -> [w21 _ _ _]
    tunnel: "Current source K6221 VISA Device 2" -> [w19 _ _ w471]
    tunnel: "Nanovoltmeter 2182a VISA Device 2" -> [w18 _ _ _]
    tunnel: "Measure two devices?" -> [w13 _ _ _]
    frame #0 {
      w24 = "Vector Angle (q)"  # Vector Angle (q)
      w25 = "\t"
      n5 = flat-sequence {
        tunnel: w22 -> [w97]
        tunnel: [w95] -> w23
        tunnel: w23 -> [w100]
        tunnel: [w98] -> w20
        tunnel: w21 -> [w102]
        tunnel: w20 -> [w108]
        frame #0 {
          n6 = call "Set-I_K6221_VISA_EL.vi"("Set I (A)"=0.0, "K6221 VISA"=w97) -> ("K6221 VISA out"=w95:refnum<visa-resource-name>)  [unwired: 2 in, 1 out]
        }
        frame #1 {
          n7 = call "KE622x -- Set Output State.vi"("Resource In"=w100, "Output State"=1) -> ("Resource Out (dupl)"=w98:refnum<visa-resource-name>)  [unwired: 12 in, 1 out]
        }
        frame #2 {
          n8 = Wait (ms)(milliseconds to wait=100) -> ()  [unwired: 1 out]
        }
        frame #3 {
          n9 = for {
            N: 5 ("Numeric") -> [_]
            tunnel: w102 -> [w104]
            w106 = u16 1 items=["Slow", "Med", "Fast"] ("Rate (NPLC)")
            w107 = FALSE ("Auto range?")
            n10 = call "Initialize_K2182A_VISA_PK.vi"("VISA address"=w104, "Auto range?"=TRUE, "Analog LPass\nFilter?"=w107, "DC\nFilter?"=w107, "Rate (NPLC)"=w106) -> ()  [unwired: 2 in]
          }
        }
        frame #4 {
          n11 = call "Set-Vcompliance_K6221_VISA_EL.vi"("Set Compliance voltage (V)"="Set Compliance voltage (V)", "K6221 VISA"=w108) -> ()  [unwired: 2 in, 2 out]
        }
      }
      n12 = case shown="True" w13 {
        tunnel: w19 -> [_ w78]
        tunnel: w18 -> [_ w77]
        frame False {
        }
        frame True {
          n13 = flat-sequence {
            tunnel: w78 -> [w82]
            tunnel: [w80] -> w79
            tunnel: w79 -> [w85]
            tunnel: [w83] -> w76
            tunnel: w77 -> [w87]
            tunnel: w76 -> [w93]
            frame #0 {
              n14 = call "Set-I_K6221_VISA_EL.vi"("Set I (A)"=0.0, "K6221 VISA"=w82) -> ("K6221 VISA out"=w80:refnum<visa-resource-name>)  [unwired: 2 in, 1 out]
            }
            frame #1 {
              n15 = call "KE622x -- Set Output State.vi"("Resource In"=w85, "Output State"=1) -> ("Resource Out (dupl)"=w83:refnum<visa-resource-name>)  [unwired: 12 in, 1 out]
            }
            frame #2 {
              n16 = Wait (ms)(milliseconds to wait=100) -> ()  [unwired: 1 out]
            }
            frame #3 {
              n17 = for {
                N: 5 ("Numeric") -> [_]
                tunnel: w87 -> [w89]
                w91 = u16 1 items=["Slow", "Med", "Fast"] ("Rate (NPLC)")
                w92 = FALSE ("Auto range?")
                n18 = call "Initialize_K2182A_VISA_PK.vi"("VISA address"=w89, "Auto range?"=TRUE, "Analog LPass\nFilter?"=w92, "DC\nFilter?"=w92, "Rate (NPLC)"=w91) -> ()  [unwired: 2 in]
              }
            }
            frame #4 {
              n19 = call "Set-Vcompliance_K6221_VISA_EL.vi"("Set Compliance voltage (V)"="Set Compliance voltage (V) 2", "K6221 VISA"=w93) -> ()  [unwired: 2 in, 2 out]
            }
          }
        }
      }
      n20 = case shown="True" w13 {
        tunnel: [FALSE w44] -> w16
        tunnel: "Folder" -> [_ w43]
        frame False {
        }
        frame True {
          w45 = "Vector Angle (q)"  # Vector Angle (q)
          w46 = "\t"
          n21 = Concatenate Strings("File name 2", ".dat" ("string")) -> (w56:string)
          n22 = String To Path(string=w56) -> (path=w50:path)
          n23 = Build Path(base path=w43, name or relative path=w50) -> (appended path=w49:path)
          n24 = Concatenate Strings("Magnetic Field Vector magnitude (T)", w46, w45, w46, "Current (A)" ("string"), w46, "Voltage (V)" ("string"), w46, "Resistance (ohm)" ("string"), w46, "Time (s)", "\r\n") -> (w57:string)
          n25 = flat-sequence {
            tunnel: w49 -> [w65]
            tunnel: w57 -> [w67]
            tunnel: [w67] -> w59
            tunnel: [w66] -> w60
            tunnel: [w61] -> w44
            tunnel: w60 -> [w73]
            tunnel: w59 -> [w74]
            frame #0 {
              n26 = Open/Create/Replace File(file path (use dialog)=w65, operation (0:open)=T1."create") -> (error out=w64:errorcluster)  [unwired: 4 in, 2 out]
              n27 = Unbundle By Name(w64) -> ("status"=w62:bool)
              n28 = case shown="True" w62 {
                tunnel: [FALSE ("Yes") w71] -> w61
                tunnel: [w68 w70] -> w66
                tunnel: w65 -> [w68 w70]
                frame False {
                }
                frame True {
                  n29 = call "Message to User2"() -> ("Yes"=w72:bool)  [unwired: 10 in, 1 out]
                  n30 = Not(x=w72) -> (.not. x?=w71:bool)
                }
              }
            }
            frame #1 {
              n31 = call <vilib>:"Write Characters To File.vi"("append to file? (new file:F)"=TRUE, "character string"=w74, "file path (dialog if empty)"=w73) -> ()  [unwired: 2 in, 1 out]
              "File path 2" <- w73
            }
          }
        }
      }
      n32 = Concatenate Strings("File name 1", ".dat" ("string")) -> (w37:string)
      n33 = String To Path(string=w37) -> (path=w31:path)
      n34 = Build Path(base path="Folder", name or relative path=w31) -> (appended path=w30:path)
      n35 = Concatenate Strings("Magnetic Field Vector magnitude (T)", w25, w24, w25, "Current (A)" ("string"), w25, "Voltage (V)" ("string"), w25, "Resistance (ohm)" ("string"), w25, "Time (s)", "\r\n") -> (w38:string)
      n36 = flat-sequence {
        tunnel: w30 -> [w113]
        tunnel: w38 -> [w116]
        tunnel: [w116] -> w41
        tunnel: [w115] -> w17
        tunnel: [w114] -> w40
        tunnel: w41 -> [w123]
        tunnel: w40 -> [w122]
        tunnel: w29 -> [w126]
        tunnel: w26 -> [w131]
        frame #0 {
          n37 = Open/Create/Replace File(file path (use dialog)=w113, operation (0:open)=T1."create") -> (error out=w112:errorcluster)  [unwired: 4 in, 2 out]
          n38 = Unbundle By Name(w112) -> ("status"=w110:bool)
          n39 = case shown="True" w110 {
            tunnel: [FALSE ("Yes") w120] -> w115
            tunnel: [w117 w119] -> w114
            tunnel: w113 -> [w117 w119]
            frame False {
            }
            frame True {
              n40 = call "Message to User"() -> ("Yes"=w121:bool)  [unwired: 10 in, 1 out]
              n41 = Not(x=w121) -> (.not. x?=w120:bool)
            }
          }
        }
        frame #1 {
          n42 = call <vilib>:"Write Characters To File.vi"("append to file? (new file:F)"=TRUE, "character string"=w123, "file path (dialog if empty)"=w122) -> ()  [unwired: 2 in, 1 out]
          "File path 1" <- w122
        }
        frame #2 {
          n43 = Concatenate Strings("CONFigure:RAMP:RATE:FIELD 1," ("String"), "Y-axis Field ramp rate (T/min)", ",3.0") -> (w127:string)
          n44 = call "430_TCP_Command.vi"("Command"=w127, "connection ID"=w126) -> ("connection ID out"=w130:refnum<k5>)  [unwired: 2 in, 2 out]
          n45 = call "430_TCP_Close.vi"("connection ID"=w130) -> ()  [unwired: 1 in, 2 out]
        }
        frame #3 {
          n46 = Concatenate Strings("CONFigure:RAMP:RATE:FIELD 1," ("String"), "Z-axis Field ramp rate (T/min)", ",9.0") -> (w133:string)
          n47 = call "430_TCP_Command.vi"("Command"=w133, "connection ID"=w131) -> ("connection ID out"=w136:refnum<k5>)  [unwired: 2 in, 2 out]
          n48 = call "430_TCP_Close.vi"("connection ID"=w136) -> ()  [unwired: 1 in, 2 out]
        }
      }
      n49 = Or(x=w17, y=w16) -> (x .or. y?=w15:bool)
      n50 = Stop(stop? (T)=w15) -> ()
    }
    frame #1 {
      n51 = flat-sequence {
        frame #0 {
          n52 = Wait (ms)(milliseconds to wait=u32 1000) -> ()  [unwired: 1 out]
        }
      }
    }
    frame #2 {
      n53 = for {
        tunnel: w141 -> [w146]
        tunnel: "From 2" -> [w145] mode=indexing
        tunnel: "To 2" -> [w144] mode=indexing
        tunnel: "Step 2" -> [w143] mode=indexing
        n54 = call "Build_serie_EL.vi"("end value"=w144, "increment"=w143, "start value"=w145) -> ("output array"=w142:dbl[])
        n55 = for {
          tunnel: w146 -> [w148]
          tunnel: w142 -> [w147] mode=indexing
          n56 = for {
            tunnel: "From" -> [w161] mode=indexing
            tunnel: "To" -> [w159] mode=indexing
            tunnel: "Step" -> [w160] mode=indexing
            tunnel: w148 -> [w158]
            tunnel: w147 -> [w153]
            n57 = flat-sequence {
              tunnel: w158 -> [w163]
              tunnel: w159 -> [w164]
              tunnel: w160 -> [w165]
              tunnel: w161 -> [w166]
              tunnel: [w166] -> w157
              tunnel: [w165] -> w156
              tunnel: [w164] -> w155
              tunnel: [w163] -> w154
              tunnel: w153 -> [w162]
              tunnel: [w162] -> w152
              tunnel: w157 -> [w172]
              tunnel: w156 -> [w171]
              tunnel: w155 -> [w170]
              tunnel: w154 -> [w168]
              tunnel: w152 -> [w167]
              frame #0 {
              }
              frame #1 {
                n58 = call "Build_serie_EL.vi"("end value"=w170, "increment"=w171, "start value"=w172) -> ("output array"=w169:dbl[])
                n59 = for {
                  tunnel: w169 -> [w186] mode=indexing
                  tunnel: w168 -> [w185]
                  tunnel: w167 -> [w184]
                  n60 = flat-sequence {
                    tunnel: [w189] -> w183
                    tunnel: [w190] -> w182
                    tunnel: w184 -> [w187]
                    tunnel: w186 -> [w188]
                    tunnel: w183 -> [w207]
                    tunnel: [w207] -> w179
                    tunnel: [w206] -> w181
                    tunnel: w182 -> [w206]
                    tunnel: [w205] -> w177
                    tunnel: [w204] -> w176
                    tunnel: [w203] -> w175
                    tunnel: [w202] -> w174
                    tunnel: w181 -> [w221]
                    tunnel: [w221] -> w180
                    tunnel: w179 -> [w220]
                    tunnel: [w220] -> w178
                    tunnel: w177 -> [w215]
                    tunnel: w176 -> [w214]
                    tunnel: w175 -> [w213]
                    tunnel: w174 -> [w212]
                    tunnel: [w211] -> w173
                    tunnel: w180 -> [w274]
                    tunnel: w178 -> [w268]
                    tunnel: w185 -> [w275]
                    tunnel: w173 -> [w262]
                    frame #0 {
                      n61 = local read "Z-axis Field ramp rate (T/min)"() -> (w198:string)
                      n62 = local read "Y-axis Field ramp rate (T/min)"() -> (w199:string)
                      n63 = local read "Magnet IP Address Z-axis"() -> (w201:string)
                      n64 = local read "Magnet IP Address Y-axis"() -> (w200:string)
                      n65 = call "Set2D_Magneticfield(polar)_PK.vi"("Y-axis Ramp Rate (T/min)"=w199, "Z-axis Ramp Rate (T/min)"=w198, "Set target vector angle (degrees)"=w188, "Set target vector magnitude (T)"=w187, "Y-Axis Magnet IP Address"=w200, "Z-Axis Magnet IP Address"=w201) -> ("Z-axis Magnetic Field (T)"=w195:string, "Y-axis Magnetic Field (T)"=w197:string, "q - Vector angle"=w190:dbl, "R - Vector field magnitude (T)"=w189:dbl)  [unwired: 2 in]
                      "Z-axis Magnetic Field (T)" <- w195
                      "Y-axis Magnetic Field (T)" <- w197
                      "Magnetic Field Vector magnitude (T)" <- w189
                      "Magnetic Field Vector Angle" <- w190
                      n66 = Build Array(w190) -> (w191:dbl[])
                      n67 = Build Array(w189) -> (w192:dbl[])
                      n68 = Fract/Exp String To Number(string=w197) -> (number=→"Y-Axis (0deg)":dbl)  [unwired: 3 in, 1 out]
                      n69 = Fract/Exp String To Number(string=w195) -> (number=→"Z-axis (90 deg)":dbl)  [unwired: 3 in, 1 out]
                      n70 = call-poly <vilib>:"Plot Helper.vi"("radius vector"=w192, "theta vector"=w191) -> ("2D Plot Class Obj Array out"=→"2D Compass":refnum<class "2D Plot Datatype.lvclass">[])  [unwired: 2 in, 7 out]
                    }
                    frame #1 {
                      n71 = local read "Nanovoltmeter 2182a VISA Device 2"() -> (w202:refnum<visa-resource-name>)
                      n72 = local read "Current source K6221 VISA Device 1"() -> (w205:refnum<visa-resource-name>)
                      n73 = local read "Current source K6221 VISA Device 2"() -> (w203:refnum<visa-resource-name>)
                      n74 = local read "Nanovoltmeter 2182a VISA Device1"() -> (w204:refnum<visa-resource-name>)
                      n75 = Multiply(x="Magnetic field stabilization time (s)", y=1000) -> (x*y=w209:dbl)
                      n76 = Wait (ms)(milliseconds to wait=w209) -> ()  [unwired: 1 out]
                    }
                    frame #2 {
                      n77 = flat-sequence {
                        tunnel: w215 -> [w247]
                        tunnel: [w245] -> w219
                        tunnel: w219 -> [w250]
                        tunnel: [w248] -> w218
                        tunnel: w218 -> [w251]
                        tunnel: [w251] -> w217
                        tunnel: w217 -> [w254]
                        tunnel: [w254] -> w216
                        tunnel: w214 -> [w253]
                        tunnel: w216 -> [w260]
                        frame #0 {
                          n78 = call "Set-I_K6221_VISA_EL.vi"("Set I (A)"=0.0, "K6221 VISA"=w247) -> ("K6221 VISA out"=w245:refnum<visa-resource-name>)  [unwired: 2 in, 1 out]
                        }
                        frame #1 {
                          n79 = call "KE622x -- Set Output State.vi"("Resource In"=w250, "Output State"=1) -> ("Resource Out (dupl)"=w248:refnum<visa-resource-name>)  [unwired: 12 in, 1 out]
                        }
                        frame #2 {
                          n80 = Wait (ms)(milliseconds to wait=100) -> ()  [unwired: 1 out]
                        }
                        frame #3 {
                          n81 = for {
                            N: 5 ("Numeric") -> [_]
                            tunnel: w253 -> [w256]
                            w258 = u16 1 items=["Slow", "Med", "Fast"] ("Rate (NPLC)")
                            w259 = FALSE ("Auto range?")
                            n82 = call "Initialize_K2182A_VISA_PK.vi"("VISA address"=w256, "Auto range?"=TRUE, "Analog LPass\nFilter?"=w259, "DC\nFilter?"=w259, "Rate (NPLC)"=w258) -> ()  [unwired: 2 in]
                          }
                        }
                        frame #4 {
                          n83 = local read "Set Compliance voltage (V)"() -> (w261:dbl)
                          n84 = call "Set-Vcompliance_K6221_VISA_EL.vi"("Set Compliance voltage (V)"=w261, "K6221 VISA"=w260) -> ()  [unwired: 2 in, 2 out]
                        }
                      }
                      n85 = local read "Measure two devices?"() -> (w211:bool)
                      n86 = case shown="True" w211 {
                        tunnel: w213 -> [_ w223]
                        tunnel: w212 -> [_ w222]
                        frame False {
                        }
                        frame True {
                          n87 = flat-sequence {
                            tunnel: w223 -> [w230]
                            tunnel: [w228] -> w227
                            tunnel: w227 -> [w233]
                            tunnel: [w231] -> w226
                            tunnel: w226 -> [w234]
                            tunnel: [w234] -> w225
                            tunnel: w225 -> [w237]
                            tunnel: [w237] -> w224
                            tunnel: w222 -> [w236]
                            tunnel: w224 -> [w243]
                            frame #0 {
                              n88 = call "Set-I_K6221_VISA_EL.vi"("Set I (A)"=0.0, "K6221 VISA"=w230) -> ("K6221 VISA out"=w228:refnum<visa-resource-name>)  [unwired: 2 in, 1 out]
                            }
                            frame #1 {
                              n89 = call "KE622x -- Set Output State.vi"("Resource In"=w233, "Output State"=1) -> ("Resource Out (dupl)"=w231:refnum<visa-resource-name>)  [unwired: 12 in, 1 out]
                            }
                            frame #2 {
                              n90 = Wait (ms)(milliseconds to wait=100) -> ()  [unwired: 1 out]
                            }
                            frame #3 {
                              n91 = for {
                                N: 5 ("Numeric") -> [_]
                                tunnel: w236 -> [w239]
                                w241 = u16 1 items=["Slow", "Med", "Fast"] ("Rate (NPLC)")
                                w242 = FALSE ("Auto range?")
                                n92 = call "Initialize_K2182A_VISA_PK.vi"("VISA address"=w239, "Auto range?"=TRUE, "Analog LPass\nFilter?"=w242, "DC\nFilter?"=w242, "Rate (NPLC)"=w241) -> ()  [unwired: 2 in]
                              }
                            }
                            frame #4 {
                              n93 = local read "Set Compliance voltage (V) 2"() -> (w244:dbl)
                              n94 = call "Set-Vcompliance_K6221_VISA_EL.vi"("Set Compliance voltage (V)"=w244, "K6221 VISA"=w243) -> ()  [unwired: 2 in, 2 out]
                            }
                          }
                        }
                      }
                    }
                    frame #3 {
                      n95 = case shown="True" w262 {
                        tunnel: "From 4" -> [_ w280]
                        tunnel: "To 4" -> [_ w279]
                        tunnel: "Step 4" -> [_ w278]
                        tunnel: cluster{dbl, "Field Reading":dbl}[] [] -> [_ w277]
                        tunnel: cluster{dbl, "Field Reading":dbl}[] [] -> [_ w276]
                        frame False {
                        }
                        frame True {
                          n96 = for {
                            tunnel: w280 -> [w287] mode=indexing
                            tunnel: w279 -> [w286] mode=indexing
                            tunnel: w278 -> [w285] mode=indexing
                            shift-right: [w282] -> _
                            shift-left: w277 -> [w284]
                            shift-right: [w281] -> _
                            shift-left: w276 -> [w283]
                            n97 = call "Build_serie_EL.vi"("end value"=w286, "increment"=w285, "start value"=w287) -> ("output array"=w288:dbl[])
                            n98 = local read "Nanovoltmeter 2182a VISA Device 2"() -> (w289:refnum<visa-resource-name>)
                            n99 = local read "Current source K6221 VISA Device 2"() -> (w290:refnum<visa-resource-name>)
                            n100 = for {
                              tunnel: w288 -> [w296] mode=indexing
                              shift-right: [w292] -> w281
                              shift-left: w283 -> [w298]
                              shift-right: [w293] -> w282
                              shift-left: w284 -> [w297]
                              tunnel: w290 -> [w295]
                              tunnel: w289 -> [w294]
                              n101 = local read "Time (s)"() -> (w291:dbl)
                              n102 = stacked-sequence {
                                tunnel: w298 -> [_ w317 _ _]
                                tunnel: [_ w318 _ _] -> w292
                                tunnel: w291 -> [_ w309 _ _]
                                tunnel: [_ w313 _ _] -> w293
                                tunnel: w297 -> [_ w311 _ _]
                                tunnel: w296 -> [w300 _ _ _]
                                tunnel: w295 -> [w299 w306 _ _]
                                tunnel: w294 -> [_ w305 _ _]
                                frame #0 {
                                n103 = flat-sequence {
                                tunnel: w300 -> [w302]
                                tunnel: w299 -> [w301]
                                frame #0 {
                                n104 = call "Set-I_K6221_VISA_EL.vi"("Set I (A)"=w302, "K6221 VISA"=w301) -> ()  [unwired: 2 in, 2 out]
                                }
                                frame #1 {
                                n105 = Wait (ms)(milliseconds to wait="wait (ms) 2") -> ()  [unwired: 1 out]
                                }
                                }
                                }
                                frame #1 {
                                n106 = local read "Number Averaging"() -> (w304:i32)
                                n107 = flat-sequence {
                                tunnel: [w323] -> w316
                                tunnel: [w328] -> w315
                                tunnel: [w325] -> w314
                                tunnel: [w327] -> w312
                                tunnel: w304 -> [w322]
                                tunnel: w311 -> [w327]
                                tunnel: w317 -> [w328]
                                tunnel: [w323] -> w310
                                tunnel: [w325] -> w308
                                tunnel: [w326] -> w307
                                tunnel: w306 -> [w320]
                                tunnel: w305 -> [w319]
                                tunnel: w316 -> [w352]
                                tunnel: [w360] -> w318
                                tunnel: w315 -> [w359]
                                tunnel: w314 -> [w351]
                                tunnel: w309 -> [w357]
                                tunnel: [w354] -> w313
                                tunnel: w312 -> [w353]
                                tunnel: w310 -> [w355]
                                tunnel: w309 -> [w350]
                                tunnel: w308 -> [w349]
                                tunnel: w307 -> [w348]
                                frame #0 {
                                n108 = for {
                                N: w322 -> [_]
                                tunnel: [w330] -> w321 mode=indexing
                                tunnel: [w329] -> w324 mode=indexing
                                tunnel: w320 -> [w335]
                                tunnel: w319 -> [w336]
                                n109 = flat-sequence {
                                tunnel: w335 -> [w337]
                                tunnel: w336 -> [w339]
                                tunnel: [w339] -> w334
                                tunnel: [w338] -> w333
                                tunnel: w334 -> [w342]
                                tunnel: w333 -> [w341]
                                tunnel: [w342] -> w332
                                tunnel: [w341] -> w331
                                tunnel: [w345] -> w329
                                tunnel: w332 -> [w344]
                                tunnel: w331 -> [w345]
                                tunnel: [w343] -> w330
                                frame #0 {
                                n110 = call "KE622x -- Get Current Level.vi"("Resource In"=w337) -> ("Current Level (A)"=w338:T2)  [unwired: 12 in, 2 out]
                                }
                                frame #1 {
                                n111 = Wait (ms)(milliseconds to wait=50) -> ()  [unwired: 1 out]
                                }
                                frame #2 {
                                n112 = call "Get-V_K2182A_VISA_EL.vi"("VISA K2182A"=w344) -> ("V (V)"=w343:dbl)  [unwired: 2 in, 2 out]
                                }
                                }
                                }
                                n113 = call "Array averaging_PK.vi"("Number averaging"=w322, "numeric array"=w321) -> ("Average value"=w323:dbl)  [unwired: 9 in]
                                "Vmeas (V) 2" <- w323
                                n114 = call "Array averaging_PK.vi"("Number averaging"=w322, "numeric array"=w324) -> ("Average value"=w325:dbl)  [unwired: 9 in]
                                "Iset (A) 2" <- w325
                                n115 = Divide(x=w323, y=w325) -> (x/y=w326:dbl)
                                "Resistance (ohm) 2" <- w326
                                }
                                frame #1 {
                                n116 = Bundle("Time (s)"=w350, "Average value"=w355) -> (w356:cluster{"Time (s)":dbl, "Average value":dbl})  [unwired: 1 in]
                                n117 = Bundle("Average value"=w349, "Average value"=w355) -> (w358:T3)  [unwired: 1 in]
                                n118 = local read "Magnetic Field Vector magnitude (T)"() -> (w347:dbl)
                                n119 = Build Array (concatenate)(w353, w356) -> (w354:cluster{"Time (s)":dbl, "Average value":dbl}[])
                                n120 = Build Array (concatenate)(w359, w358) -> (w360:T4)
                                "V vs I 2" <- w360
                                n121 = local read "Magnetic Field Vector Angle"() -> (w346:dbl)
                                n122 = Build Array(w347, w346, w351, w352, w348, w357) -> (→"data 2":dbl[])
                                }
                                }
                                }
                                frame #2 {
                                n123 = Wait (ms)(milliseconds to wait=u32 50) -> ()  [unwired: 1 out]
                                }
                                frame #3 {
                                n124 = local read "data 2"() -> (w363:dbl[])
                                n125 = local read "File path 2"() -> (w365:path)
                                n126 = Array To Spreadsheet String(array=w363, 3:"%e" ("format string")) -> (spreadsheet string=w366:string)  [unwired: 1 in]
                                n127 = call <vilib>:"Write Characters To File.vi"("append to file? (new file:F)"=TRUE, "character string"=w366, "file path (dialog if empty)"=w365) -> ()  [unwired: 2 in, 1 out]
                                }
                              }
                            }
                          }
                        }
                      }
                      n128 = for {
                        tunnel: w275 -> [w380]
                        tunnel: w268 -> [w378]
                        tunnel: w274 -> [w377]
                        tunnel: "From 3" -> [w372] mode=indexing
                        tunnel: "Step 3" -> [w371] mode=indexing
                        tunnel: "To 3" -> [w370] mode=indexing
                        shift-right: [w369] -> _
                        shift-left: cluster{dbl, "Field Reading":dbl}[] [] -> [w376]
                        shift-right: [w368] -> _
                        shift-left: cluster{dbl, "Field Reading":dbl}[] [] -> [w379]
                        n129 = call "Build_serie_EL.vi"("end value"=w370, "increment"=w371, "start value"=w372) -> ("output array"=w373:dbl[])
                        n130 = local read "Current source K6221 VISA Device 1"() -> (w375:refnum<visa-resource-name>)
                        n131 = local read "Nanovoltmeter 2182a VISA Device1"() -> (w374:refnum<visa-resource-name>)
                        n132 = for {
                          tunnel: w380 -> [w394]
                          tunnel: w378 -> [w388]
                          tunnel: w377 -> [w387]
                          tunnel: w373 -> [w385] mode=indexing
                          shift-right: [w381] -> w368
                          shift-left: w379 -> [w393]
                          shift-right: [w382] -> w369
                          shift-left: w376 -> [w386]
                          tunnel: w375 -> [w384]
                          tunnel: w374 -> [w383]
                          n133 = Tick Count (ms)() -> (millisecond timer value=w390:u32)
                          n134 = Subtract(x=w390, y=w394) -> (x-y=w392:u32)
                          n135 = Divide(x=w392, y=1000.0) -> (x/y=w389:dbl)
                          "Time (s)" <- w389
                          n136 = stacked-sequence {
                            tunnel: w393 -> [_ w416 _ _]
                            tunnel: [_ w417 _ _] -> w381
                            tunnel: w389 -> [_ w404 _ _]
                            tunnel: w388 -> [_ w411 _ _]
                            tunnel: w387 -> [_ w410 _ _]
                            tunnel: [_ w409 _ _] -> w382
                            tunnel: w386 -> [_ w407 _ _]
                            tunnel: w385 -> [w396 _ _ _]
                            tunnel: w384 -> [w395 w401 _ _]
                            tunnel: w383 -> [_ w400 _ _]
                            frame #0 {
                              n137 = flat-sequence {
                                tunnel: w396 -> [w398]
                                tunnel: w395 -> [w397]
                                frame #0 {
                                n138 = call "Set-I_K6221_VISA_EL.vi"("Set I (A)"=w398, "K6221 VISA"=w397) -> ()  [unwired: 2 in, 2 out]
                                }
                                frame #1 {
                                n139 = Wait (ms)(milliseconds to wait="wait (ms)") -> ()  [unwired: 1 out]
                                }
                              }
                            }
                            frame #1 {
                              n140 = flat-sequence {
                                tunnel: [w422] -> w415
                                tunnel: [w428] -> w414
                                tunnel: [w424] -> w413
                                tunnel: [w427] -> w412
                                tunnel: [w426] -> w408
                                tunnel: "Number Averaging" -> [w421]
                                tunnel: w407 -> [w426]
                                tunnel: w416 -> [w428]
                                tunnel: w411 -> [w427]
                                tunnel: [w422] -> w405
                                tunnel: [w424] -> w403
                                tunnel: [w425] -> w402
                                tunnel: w401 -> [w419]
                                tunnel: w400 -> [w418]
                                tunnel: w415 -> [w450]
                                tunnel: [w460] -> w417
                                tunnel: w414 -> [w459]
                                tunnel: w413 -> [w449]
                                tunnel: w412 -> [w454]
                                tunnel: w404 -> [w457]
                                tunnel: w410 -> [w456]
                                tunnel: [w452] -> w409
                                tunnel: w408 -> [w451]
                                tunnel: w405 -> [w453]
                                tunnel: w404 -> [w448]
                                tunnel: w403 -> [w447]
                                tunnel: w402 -> [w446]
                                frame #0 {
                                n141 = for {
                                N: w421 -> [_]
                                tunnel: [w430] -> w420 mode=indexing
                                tunnel: [w429] -> w423 mode=indexing
                                tunnel: w419 -> [w435]
                                tunnel: w418 -> [w436]
                                n142 = flat-sequence {
                                tunnel: w435 -> [w437]
                                tunnel: w436 -> [w439]
                                tunnel: [w439] -> w434
                                tunnel: [w438] -> w433
                                tunnel: w434 -> [w442]
                                tunnel: w433 -> [w441]
                                tunnel: [w442] -> w432
                                tunnel: [w441] -> w431
                                tunnel: [w445] -> w429
                                tunnel: w432 -> [w444]
                                tunnel: w431 -> [w445]
                                tunnel: [w443] -> w430
                                frame #0 {
                                n143 = call "KE622x -- Get Current Level.vi"("Resource In"=w437) -> ("Current Level (A)"=w438:T2)  [unwired: 12 in, 2 out]
                                }
                                frame #1 {
                                n144 = Wait (ms)(milliseconds to wait=50) -> ()  [unwired: 1 out]
                                }
                                frame #2 {
                                n145 = call "Get-V_K2182A_VISA_EL.vi"("VISA K2182A"=w444) -> ("V (V)"=w443:dbl)  [unwired: 2 in, 2 out]
                                }
                                }
                                }
                                n146 = call "Array averaging_PK.vi"("Number averaging"=w421, "numeric array"=w423) -> ("Average value"=w424:dbl)  [unwired: 9 in]
                                "Iset (A)" <- w424
                                n147 = call "Array averaging_PK.vi"("Number averaging"=w421, "numeric array"=w420) -> ("Average value"=w422:dbl)  [unwired: 9 in]
                                "Vmeas (V)" <- w422
                                n148 = Divide(x=w422, y=w424) -> (x/y=w425:dbl)
                                "Resistance (ohm)" <- w425
                                }
                                frame #1 {
                                n149 = Build Array(w454, w456, w449, w450, w446, w457) -> (→"data":dbl[])
                                n150 = Bundle(w448, "Average value"=w453) -> (w455:cluster{dbl, "Average value":dbl})  [unwired: 1 in]
                                n151 = Bundle("Average value"=w447, "Average value"=w453) -> (w458:T3)  [unwired: 1 in]
                                n152 = Build Array (concatenate)(w451, w455) -> (w452:cluster{dbl, "Average value":dbl}[])
                                n153 = Build Array (concatenate)(w459, w458) -> (w460:T4)
                                "V vs I" <- w460
                                }
                              }
                            }
                            frame #2 {
                              n154 = Wait (ms)(milliseconds to wait=u32 50) -> ()  [unwired: 1 out]
                            }
                            frame #3 {
                              n155 = local read "data"() -> (w463:dbl[])
                              n156 = Array To Spreadsheet String(array=w463, 3:"%e" ("format string")) -> (spreadsheet string=w466:string)  [unwired: 1 in]
                              n157 = local read "File path 1"() -> (w465:path)
                              n158 = call <vilib>:"Write Characters To File.vi"("append to file? (new file:F)"=TRUE, "character string"=w466, "file path (dialog if empty)"=w465) -> ()  [unwired: 2 in, 1 out]
                            }
                          }
                        }
                      }
                    }
                  }
                }
              }
              frame #2 {
                n159 = Multiply(x="Wait time after each sweep(min)", y=60000.0) -> (x*y=w470:dbl)
                n160 = Wait (ms)(milliseconds to wait=w470) -> ()  [unwired: 1 out]
              }
            }
          }
        }
      }
    }
    frame #3 {
      n161 = flat-sequence {
        tunnel: w473 -> [w482]
        tunnel: [w480] -> w474
        tunnel: w474 -> [w484]
        frame #0 {
          n162 = call "Set-I_K6221_VISA_EL.vi"("Set I (A)"=0.0, "K6221 VISA"=w482) -> ("K6221 VISA out"=w480:refnum<visa-resource-name>)  [unwired: 2 in, 1 out]
        }
        frame #1 {
          n163 = call "KE622x -- Set Output State.vi"("Resource In"=w484, "Output State"=0) -> ()  [unwired: 12 in, 2 out]
        }
      }
      n164 = flat-sequence {
        tunnel: w471 -> [w477]
        tunnel: [w475] -> w472
        tunnel: w472 -> [w479]
        frame #0 {
          n165 = call "Set-I_K6221_VISA_EL.vi"("Set I (A)"=0.0, "K6221 VISA"=w477) -> ("K6221 VISA out"=w475:refnum<visa-resource-name>)  [unwired: 2 in, 1 out]
        }
        frame #1 {
          n166 = call "KE622x -- Set Output State.vi"("Resource In"=w479, "Output State"=0) -> ()  [unwired: 12 in, 2 out]
        }
      }
    }
  }
